vi "Glide Multiplier.vi"(5 "Array in":dbl[](array[numeric]), 6 "new mult":dbl, 7 "last mult":dbl) -> (1 "Array out":dbl[](array[numeric]))   [LabVIEW 2020, in "Level.lvclass"]
uses:
  Level.lvclass
  Level.lvclass/Level.ctl
  <vilib>/Analysis/NI_AALBase.lvlib
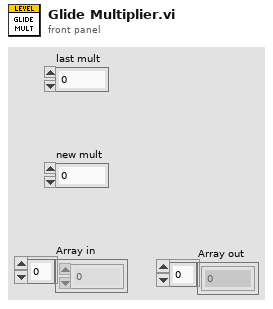
[diagram p1: front panel]
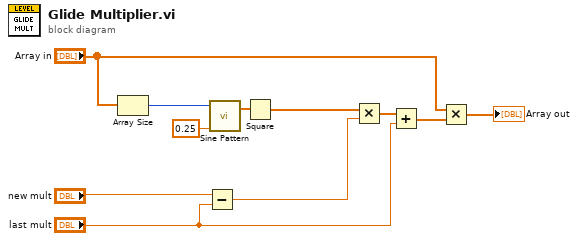
[diagram p0: block diagram]
diagram:
  n1 = Array Size(array="Array in") -> (size(s)=w9:i32)
  n2 = Subtract(x="new mult", y="last mult") -> (x-y=w5:dbl)
  n3 = call <vilib>:"Sine Pattern.vi"("cycles"=0.25, "samples"=w9) -> ("Sinusoidal Pattern"=w10:dbl[])  [unwired: 2 in, 1 out]
  n4 = Square(x=w10) -> (x^2=w7:dbl[])
  n5 = Multiply(x=w7, y=w5) -> (x*y=w8:dbl[])
  n6 = Add(x=w8, y="last mult") -> (x+y=w3:dbl[])
  n7 = Multiply(x="Array in", y=w3) -> (x*y=→"Array out":dbl[])
